vi "Robotic Arm_3.vi"() -> ()   [LabVIEW 2020]
panel:
  out "Arm":bool=TRUE
  in  "Lever":bool=TRUE
  in  "LEFT/RIGHT":dbl(slide)=461.21588594704684 scale=191.0..1000.0
  in  "stop":bool
  out "Container":bool
  in  "UP/DOWN":dbl(slide)=243.38085539714865 scale=500.0..200.0
  # "GRAB ITEM"
  # "LEAVE ITEM"
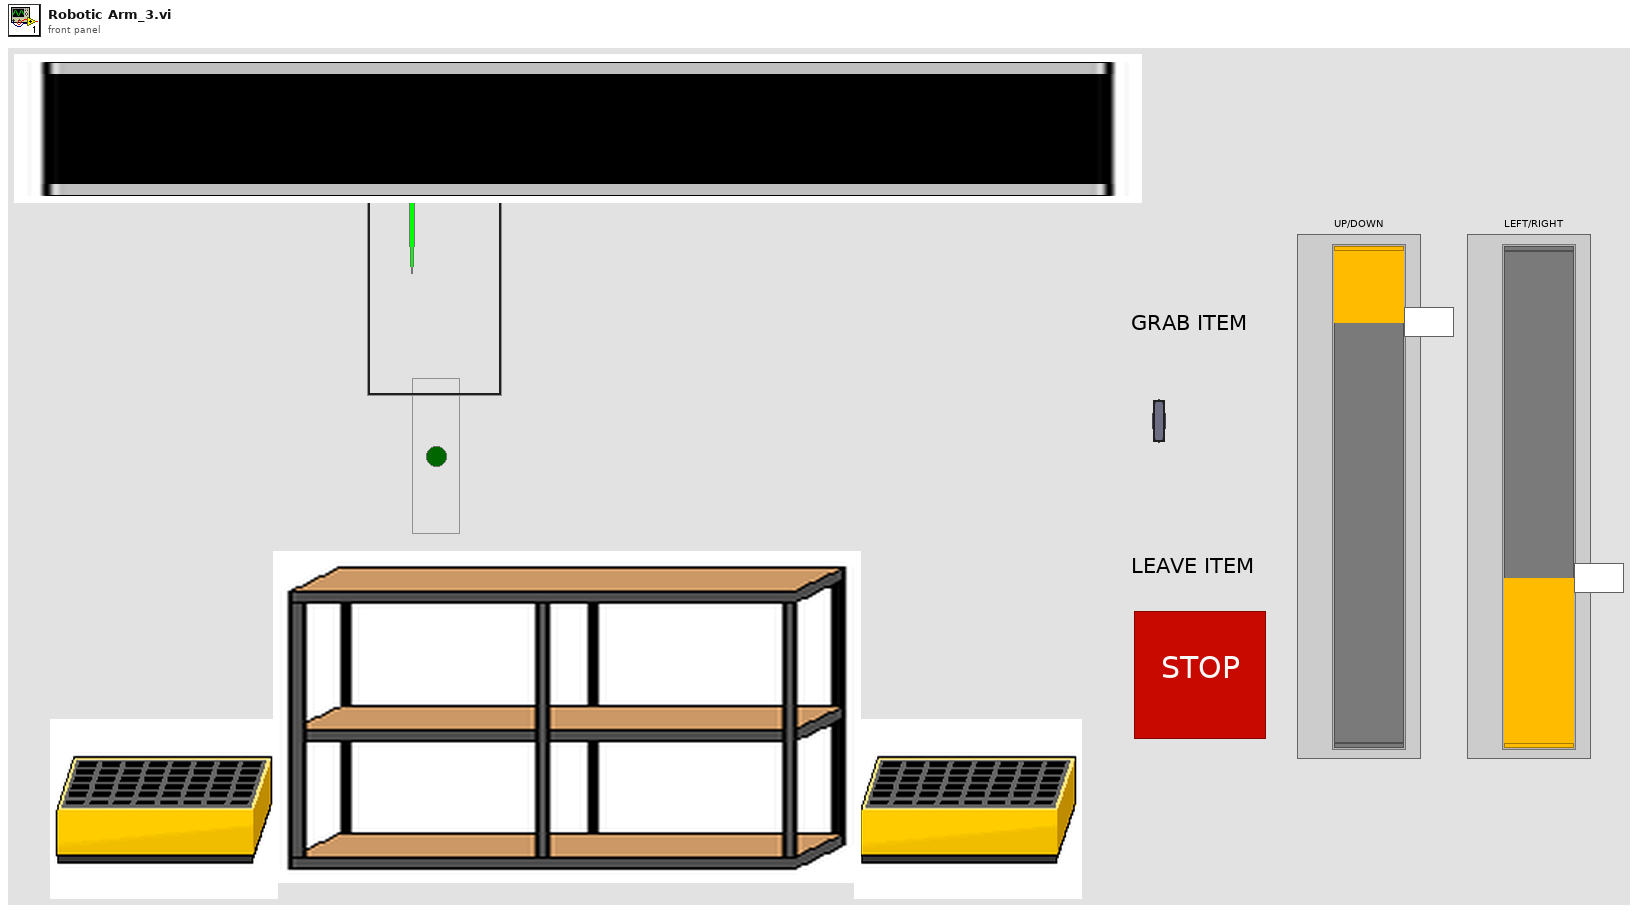
[diagram p1: front panel]
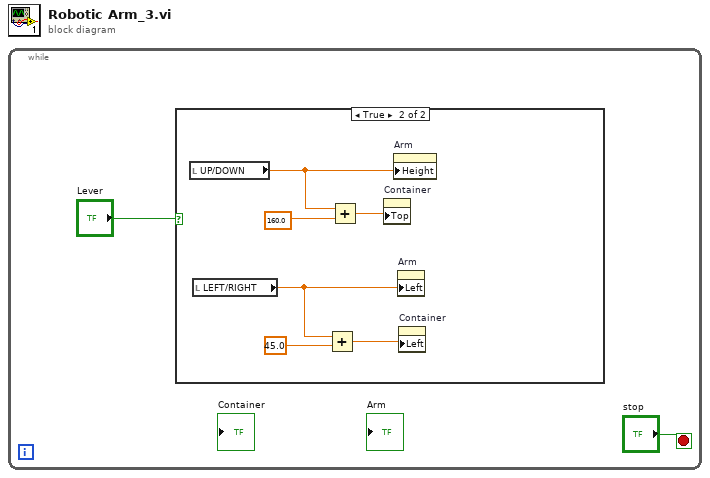
[diagram p0: block diagram]
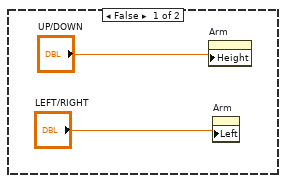
[diagram p2: hidden frame]
diagram:
  n1 = while {
    stop <- "stop" stop-if-true
    n2 = case shown="True" "Lever" {
      frame False {
        n3 = property on="Arm" class="Bool (strict)"("Height"="UP/DOWN") -> ()  [unwired: 2 in, 2 out]
        n4 = property on="Arm" class="Bool (strict)"("Left"="LEFT/RIGHT") -> ()  [unwired: 2 in, 2 out]
      }
      frame True {
        n5 = local read "UP/DOWN"() -> (w8:dbl)
        n6 = local read "LEFT/RIGHT"() -> (w6:dbl)
        n7 = Add(x=w6, y=45.0) -> (x+y=w5:dbl)
        n8 = Add(x=w8, y=160.0) -> (x+y=w9:dbl)
        n9 = property on="Container" class="Bool (strict)"("Top"=w9) -> ()  [unwired: 2 in, 2 out]
        n10 = property on="Arm" class="Bool (strict)"("Height"=w8) -> ()  [unwired: 2 in, 2 out]
        n11 = property on="Arm" class="Bool (strict)"("Left"=w6) -> ()  [unwired: 2 in, 2 out]
        n12 = property on="Container" class="Bool (strict)"("Left"=w5) -> ()  [unwired: 2 in, 2 out]
      }
    }
  }
